vi "enviar_comando2.vi"(8 "error in (no error)":errorcluster, 10 "Command":string="*IDN?") -> (0 "error out":errorcluster, 2 "Response":string, 3 "Pistofono out":refnum<class "Pistofono.lvclass">)   [LabVIEW 2019]
uses:
  Pistofono.lvclass
  <vilib>/Instr/_visa.llb/VISA Configure Serial Port (Instr).vi
panel:
  in  "Read Count":u32=1000
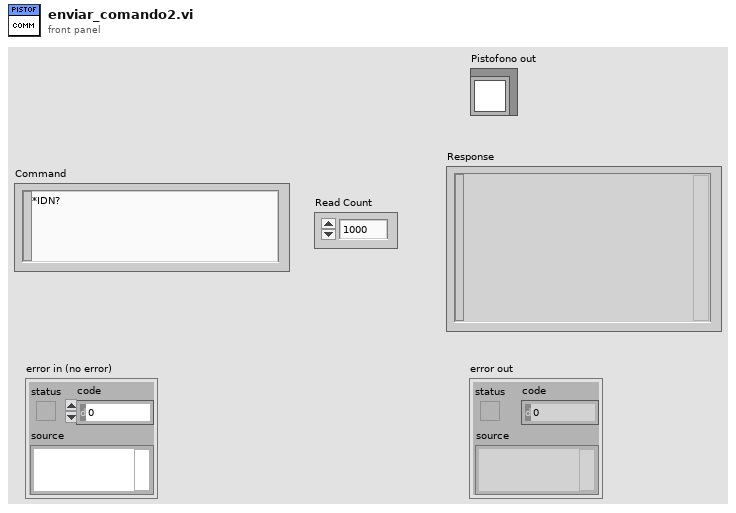
[diagram p1: front panel]
types:
  T1 = cluster{"baud rate":u32, "data bits":u16, "parity":enum16{"None", "Odd", "Even", "Mark", "Space"}, "stop bits":u16, "flow control":u16}
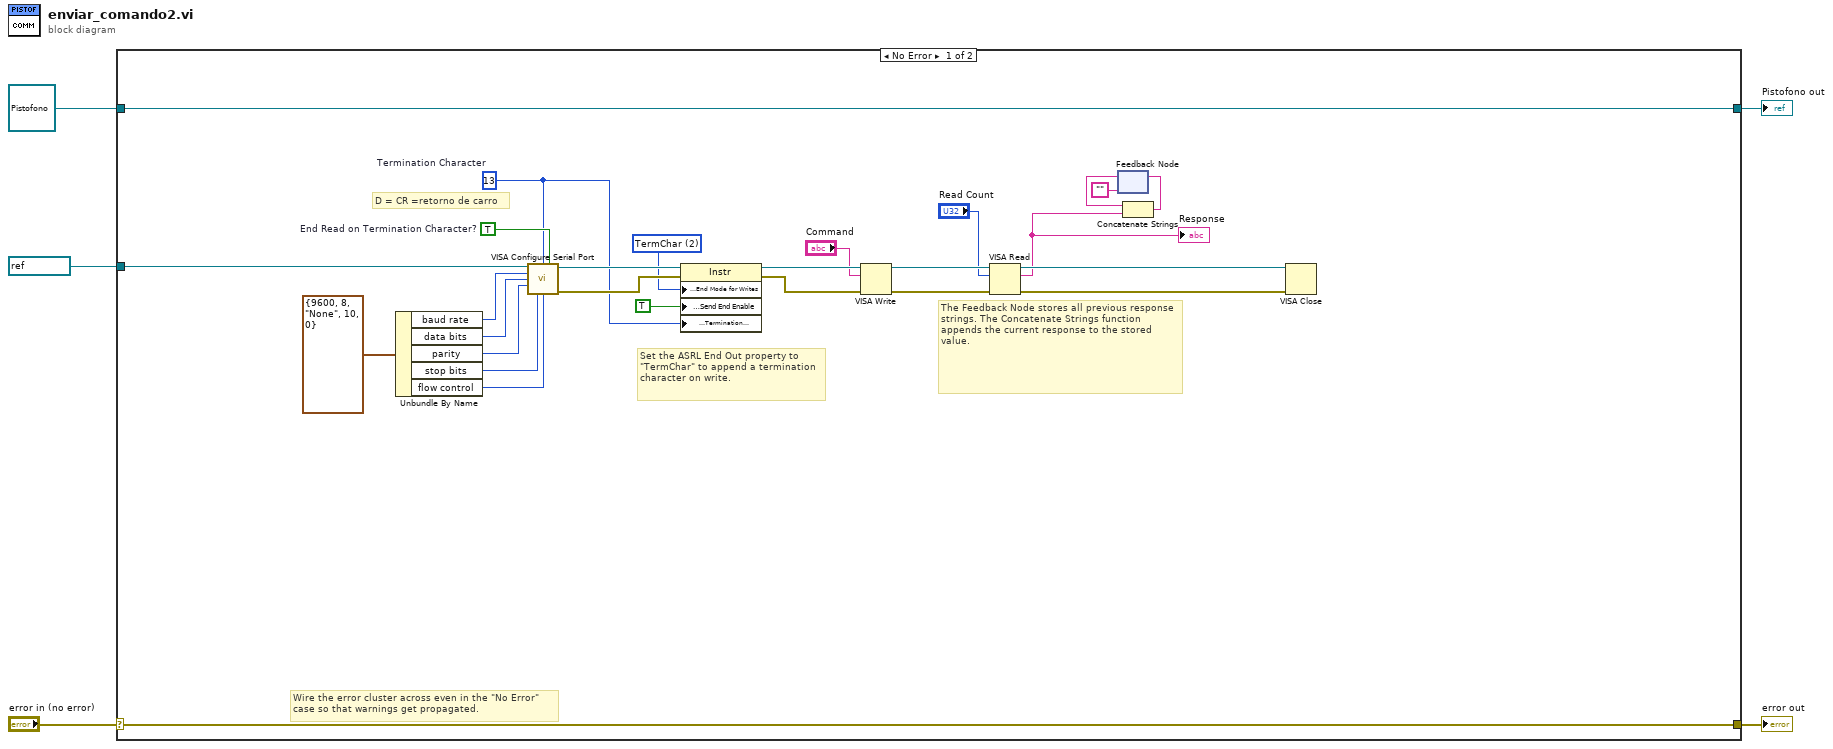
[diagram p0: block diagram]
diagram:
  n1 = case shown="No Error" "error in (no error)" {
    selector: "error in (no error)" -> [w31 w34]
    tunnel: [w31 w34] -> w4
    tunnel: [w32 w33] -> w2
    tunnel: refnum<class "Pistofono.lvclass"> refnum ("Pistofono in") -> [w32 w33]
    tunnel: refnum<visa-resource-name> "COM3" ("VISA resource name") -> [w7 _]
    frame No Error {
      w17 = u8 13  # Termination Character
      w9 = u16 2 items=["None", "LastBit", "TermChar", "Break"] ("Serial Settings:Serial End Mode for Writes")
      w23 = TRUE  # End Read on Termination Character?
      # "D = CR =retorno de carro"
      # "The Feedback Node stores all previous response strings. The Concatenate Strings function appends the current response to the stored value."
      # "Set the ASRL End Out property to \"TermChar\" to append a termination character on write."
      # "Wire the error cluster across even in the \"No Error\"\ncase so that warnings get propagated."
      n2 = Unbundle By Name(T1 {"baud rate"=9600, "data bits"=8, "parity"=enum."None", "stop bits"=10, "flow control"=0} ("Serial Settings")) -> ("baud rate"=w25:u32, "data bits"=w26:u16, "parity"=w27:enum16{"None", "Odd", "Even", "Mark", "Space"}, "stop bits"=w28:u16, "flow control"=w20:u16)
      n3 = call-poly "VISA Configure Serial Port"("VISA resource name"=w7, "termination char\n(0xA = '\\n' = LF)"=w17, "Enable Termination\nChar (T)"=w23, "baud rate (9600)"=w25, "data bits (8)"=w26, "parity (0:none)"=w27, "stop bits (10: 1 bit)"=w28, "flow control (0:none)"=w20) -> ("VISA resource name out"=w29:refnum<visa-resource-name>, "error out"=w30:errorcluster)  [unwired: 2 in, 4 out]
      n4 = property class="Instr"(reference=w29, error in=w30, "Serial Settings:End Mode for Writes"=w9, "Message Based Settings:Send End Enable"=TRUE, "Message Based Settings:Termination Character"=w17) -> (reference out=w18:refnum<visa-resource-name>, error out=w19:errorcluster)
      n5 = VISA Write(VISA resource name=w18, write buffer="Command", error in (no error)=w19) -> (VISA resource name out=w16:refnum<visa-resource-name>, error out=w15:errorcluster)  [unwired: 1 out]
      n6 = VISA Read(VISA resource name=w16, byte count="Read Count", error in (no error)=w15) -> (VISA resource name out=w21:refnum<visa-resource-name>, read buffer=w6:string, error out=w22:errorcluster)  [unwired: 1 out]
      "Response" <- w6
      n7 = feedback #1("") -> (w12:string)
      n8 = Concatenate Strings(w12, w6) -> (w11:string)
      n9 = feedback-in #1(w11) -> ()
      n10 = VISA Close(VISA resource name=w21, error in (no error)=w22) -> ()  [unwired: 1 out]
    }
    frame Error {
    }
  }
  "error out" <- w4
  "Pistofono out" <- w2
